vi "DriveStraightv2.vi"(4 "MotrSpdInfo":T1={"TrgtCounts"=0, "Accel?"=FALSE, "CurrCounts"=0.0, "SlowConst"=572.75, "MinPwr"=572.75} {"MinPwr" format="%#_13g"; "SlowConst" format="%#_13g"}, 6 "FirstTime?":bool, 7 "Sensitivity":dbl, 8 "Range":dbl, 9 "MotorPwrIn":dbl, 10 "Initial":dbl, 11 "Heading":dbl) -> (0 "RightOut":dbl, 3 "LeftOut":dbl)   [LabVIEW 2017]
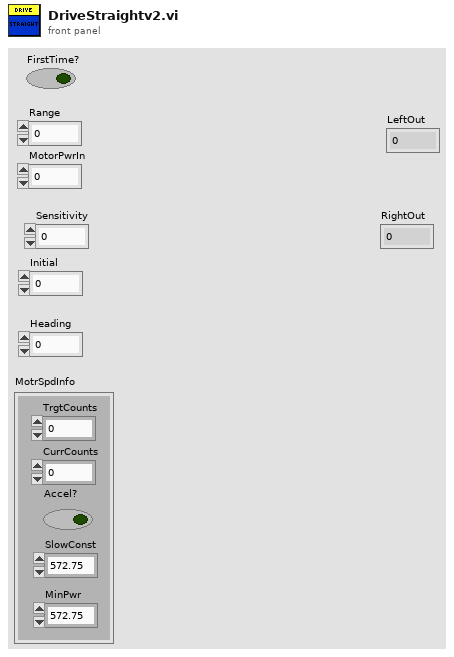
[diagram p1: front panel]
types:
  T1 = cluster{"TrgtCounts":i32, "Accel?":bool, "CurrCounts":dbl, "SlowConst":dbl, "MinPwr":dbl}
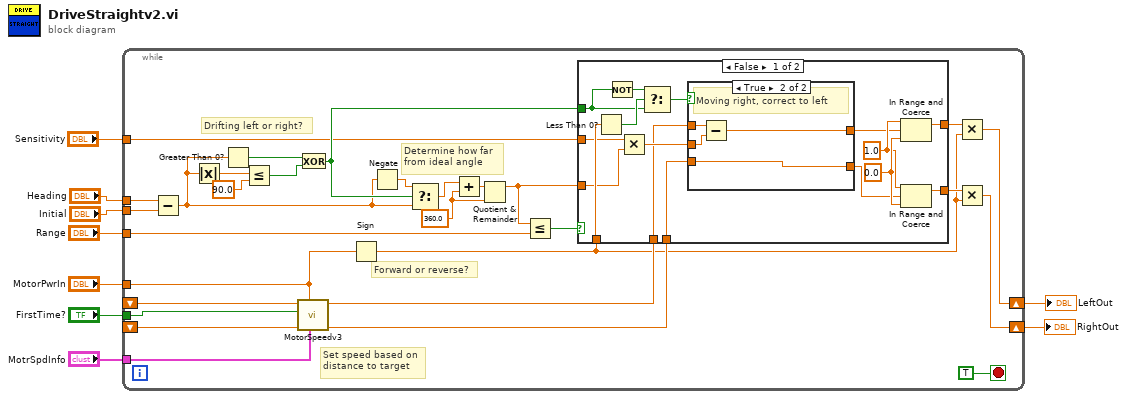
[diagram p0: block diagram]
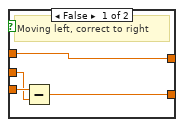
[diagram p2: hidden frame]
diagram:
  n1 = while {
    tunnel: "Heading" -> [w38]
    tunnel: "Initial" -> [w37]
    tunnel: "Range" -> [w26]
    tunnel: "Sensitivity" -> [w24]
    tunnel: "MotorPwrIn" -> [w10]
    tunnel: "FirstTime?" -> [w11]
    shift-right: [w14] -> w4
    shift-left: _ -> [w20]
    shift-right: [w13] -> w3
    shift-left: _ -> [w21]
    tunnel: "MotrSpdInfo" -> [w12]
    stop <- TRUE stop-if-true
    w30 = 360.0 ("value")
    # "Forward or reverse?"
    # "Set speed based on\ndistance to target"
    # "Determine how far\nfrom ideal angle"
    # "Drifting left or right?"
    n2 = Subtract(x=w38, y=w37) -> (x-y=w27:dbl)
    n3 = Absolute Value(x=w27) -> (abs(x)=w34:dbl)
    n4 = Greater Than 0?(x=w27) -> (x > 0?=w36:bool)
    n5 = Less Or Equal?(x=w34, y=90.0) -> (x <= y?=w35:bool)
    n6 = call "MotorSpeedv3.vi"("MotrSpdInfo"=w12, "MaxPwr"=w10, "RightSpdIn"=w20, "FirstTime?"=w11, "LeftSpdIn"=w21) -> ("RightSpdOut"=w18:dbl, "LeftSpdOut"=w19:dbl)  [unwired: 5 in]
    n7 = Exclusive Or(1:w35, 2:w36) -> (0:w28:bool)
    n8 = Sign(1:w10) -> (0:w15:dbl)
    n9 = Negate(x=w27) -> (-x=w29:dbl)
    n10 = Select(t=w29, s=w28, f=w27) -> (s? t:f=w31:dbl)
    n11 = Add(x=w31, y=w30) -> (x+y=w32:dbl)
    n12 = Quotient & Remainder(x=w32, y=w30) -> (x-y*floor(x/y)=w23:dbl)  [unwired: 1 out]
    n13 = Less Or Equal?(x=w23, y=w26) -> (x <= y?=w25:bool)
    n14 = case shown="False" w25 {
      tunnel: w28 -> [w48 _]
      tunnel: w24 -> [w42 _]
      tunnel: w23 -> [w41 _]
      tunnel: w19 -> [w44 w64]
      tunnel: [w51 w64] -> w17
      tunnel: [w50 w63] -> w16
      tunnel: w15 -> [w45 _]
      tunnel: w18 -> [w43 w63]
      frame False {
        w53 = 0.0 ("lower limit")
        w52 = 1.0 ("upper limit")
        n15 = Less Than 0?(x=w45) -> (x < 0?=w49:bool)
        n16 = Not(x=w48) -> (.not. x?=w47:bool)
        n17 = Multiply(x=w42, y=w41) -> (x*y=w54:dbl)
        n18 = Select(t=w47, s=w49, f=w48) -> (s? t:f=w46:bool)
        n19 = case shown="True" w46 {
          tunnel: w44 -> [w58 w61]
          tunnel: w54 -> [w56 w62]
          tunnel: [w55 w59] -> w40
          tunnel: [w58 w60] -> w39
          tunnel: w43 -> [w57 w59]
          frame False {
            # "Moving left, correct to right"
            n20 = Subtract(x=w57, y=w56) -> (x-y=w55:dbl)
          }
          frame True {
            # "Moving right, correct to left"
            n21 = Subtract(x=w61, y=w62) -> (x-y=w60:dbl)
          }
        }
        n22 = In Range and Coerce(upper limit=w52, x=w39, lower limit=w53) -> (coerced(x)=w51:dbl)  [unwired: 1 out]
        n23 = In Range and Coerce(upper limit=w52, x=w40, lower limit=w53) -> (coerced(x)=w50:dbl)  [unwired: 1 out]
      }
      frame True {
      }
    }
    n24 = Multiply(x=w17, y=w15) -> (x*y=w13:dbl)
    n25 = Multiply(x=w16, y=w15) -> (x*y=w14:dbl)
  }
  "LeftOut" <- w3
  "RightOut" <- w4
